vi "Initialize.vi"(8 "error in (no error)":errorcluster, 11 "MB in":refnum<class "WebSocket Client CR.lvclass">) -> (0 "error out":errorcluster, 3 "MB out":refnum<class "WebSocket Client CR.lvclass">)   [LabVIEW 2021, in "WebSockets.lvlib" / "WebSocket Client CR.lvclass"]
uses:
  WebSocket Client CR.lvclass
  WebSocket Client CR.lvclass/WebSocket Client CR.ctl
  ctl/MB timeouts.ctl
  Master CR/Param/TCP Param/TCP Param.lvclass
  Master CR/Param/TCP Param/TCP Param.lvclass/TCP Param.ctl
  WebSocket Client/WebSocket Client.lvclass
  C:/my_projects/projects/Algorithms/Labview/21/WebSockets/Source/WebSockets/WebSocket/WebSocket.lvclass
  Modbus_v121c/Data Model/Device Data Model.lvclass
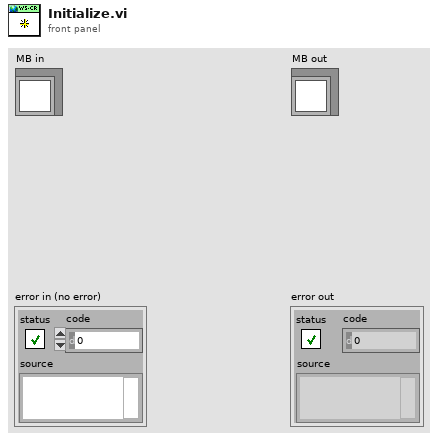
[diagram p1: front panel]
types:
  T1 = typedef "WebSockets.lvlib/WebSocket Client CR.lvclass/MB timeouts.ctl" = cluster{"reconn_timeout":i32, "N attempt max":i32, "t_reset_TTL":i32, "period":i32}
  T2 = typedef "Param.lvlib/TCP Param.lvclass/timeouts.ctl" = cluster{"conn_timeout":i32, "reconn_timeout":i32, "N attempt max":i32, "t_reset_TTL":i32, "write_timeout":i32, "read_timeout":i32, "period":i32}
  T3 = cluster{"Remote IP Address":string, "Remote Port":u16}
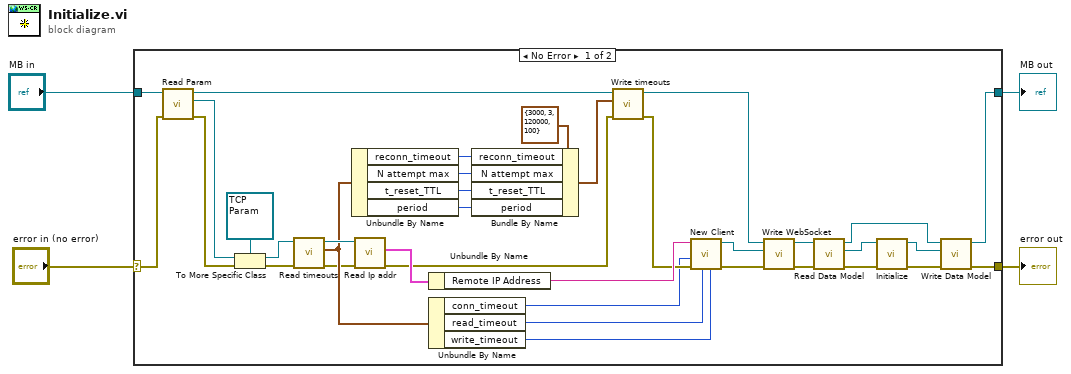
[diagram p0: block diagram]
diagram:
  n1 = case shown="No Error" "error in (no error)" {
    selector: "error in (no error)" -> [w14 w41]
    tunnel: [w34 w41] -> w3
    tunnel: [w35 w42] -> w1
    tunnel: "MB in" -> [w16 w42]
    frame No Error {
      n2 = call "Read Param.vi"("error in (no error)"=w14, "MB_TCP in"=w16) -> ("error out"=w23:errorcluster, "Param"=w21:refnum<class "Param.lvclass">, "MB_TCP out"=w20:refnum<class "WebSocket Client CR.lvclass">)  [unwired: 7 in]
      n3 = To More Specific Class(target class=refnum<class "TCP Param.lvclass"> refnum ("Param.lvlib:TCP Param.lvclass"), reference=w21, error in=w23) -> (specific class reference=w22:refnum<class "TCP Param.lvclass">, error out=w32:errorcluster)
      n4 = call "Read timeouts.vi"("error in (no error)"=w32, "MBParam in"=w22) -> ("error out"=w18:errorcluster, "timeouts"=w19:T2, "MBParam out"=w25:refnum<class "TCP Param.lvclass">)  [unwired: 7 in]
      n5 = Unbundle By Name(w19) -> ("reconn_timeout"=w30:i32, "N attempt max"=w27:i32, "t_reset_TTL"=w28:i32, "period"=w29:i32)
      n6 = call "Read Ip addr.vi"("error in (no error)"=w18, "MBParam in"=w25) -> ("error out"=w17:errorcluster, "IP address"=w24:T3)  [unwired: 7 in, 1 out]
      n7 = Unbundle By Name(w24) -> ("Remote IP Address"=w11:string)
      n8 = Unbundle By Name(w19) -> ("conn_timeout"=w9:i32, "read_timeout"=w8:i32, "write_timeout"=w7:i32)
      n9 = Bundle By Name(cluster=T1 {"reconn_timeout"=3000, "N attempt max"=3, "t_reset_TTL"=120000, "period"=100} ("MB timeouts"), "reconn_timeout"=w30, "N attempt max"=w27, "t_reset_TTL"=w28, "period"=w29) -> (w26:T1)
      n10 = call "Write timeouts.vi"("error in (no error)"=w17, "MB timeouts"=w26, "Master CR in"=w20) -> ("error out"=w10:errorcluster, "Master CR out"=w15:refnum<class "WebSocket Client CR.lvclass">)  [unwired: 7 in]
      n11 = call "New Client.vi"("write operation timeout"=w7, "read operation timeout"=w8, "error in (no error)"=w10, "connect timeout ms"=w9, "WebSocket URL"=w11) -> ("error out"=w5:errorcluster, "WebSocket Client out"=w6:refnum<class "WebSocket Client.lvclass">)  [unwired: 5 in]
      n12 = call "Write WebSocket.vi"("error in (no error)"=w5, "WebSocket"=w6, "Master CR in"=w15) -> ("error out"=w12:errorcluster, "Master CR out"=w13:refnum<class "WebSocket Client CR.lvclass">)  [unwired: 7 in]
      n13 = call "Read Data Model.vi"("error in (no error)"=w12, "Master CR in"=w13) -> ("error out"=w39:errorcluster, "Data Model"=w40:refnum<class "Device Data Model.lvclass">, "Master CR out"=w36:refnum<class "WebSocket Client CR.lvclass">)  [unwired: 7 in]
      n14 = call-dynamic "Initialize.vi"("error in"=w39, "device data model in"=w40) -> ("error out"=w38:errorcluster, "device data model out"=w37:refnum<class "Device Data Model.lvclass">)  [unwired: 8 in]
      n15 = call "Write Data Model.vi"("error in (no error)"=w38, "Data Model"=w37, "Master CR in"=w36) -> ("error out"=w34:errorcluster, "Master CR out"=w35:refnum<class "WebSocket Client CR.lvclass">)  [unwired: 7 in]
    }
    frame Error {
    }
  }
  "error out" <- w3
  "MB out" <- w1
